vi "rs3 init devices_and_sensors.vi"(6 "rscontext":u64=1752067024, 8 "error in":errorcluster, 9 "api_version":i32=20710, 10 "Select Device":i32, 11 "Select Sensor":i32) -> (0 "error out":errorcluster, 1 "Adv. enable?":i32, 2 "init results":T3, 3 "init error":string, 4 "All Devices":T2(array[cluster]), 5 "Sensor Array":T1(array[cluster]), 7 "Found RealSense":bool)   [LabVIEW 2023]
doc: "Initialized the RealSense device. \nSelect the specific DEVICE and its specific SENSOR. \n\n\nINPUT:\nSelect Device The INDEX to the specific DEVICE handle\nSelect Sensor The INDEX to the specific SENSOR that is part of the selected DEVICE.\n \nOUTPUT:\ninit result Contains all the information about the selected device and its sensor. You will need to use the Dev Out HANDLE to communicate with the device. \n \nselected sensor array Contains the arrays of SENSORS attached to a specific DEVICE.\nall devices Contains array of all device that are attached to the PC."
panel:
  # "RS3 Init Device and Sensors"
  # "(C) Intel Corp. 2017,  AGJ"
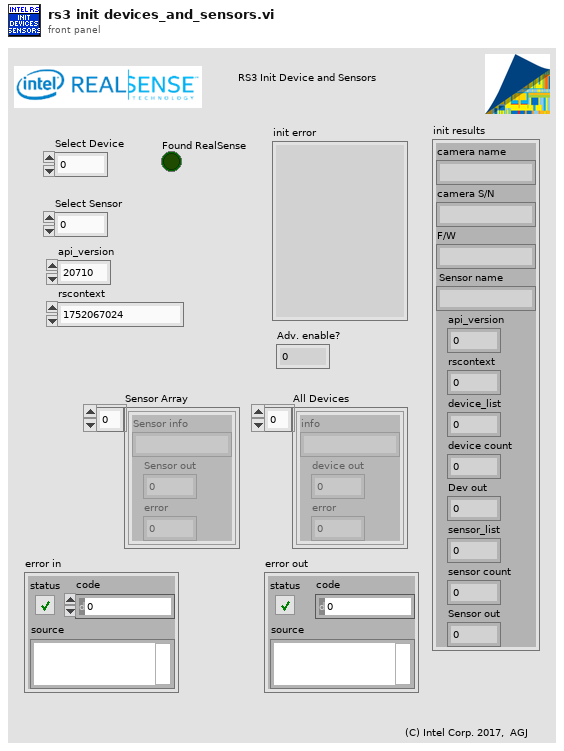
[diagram p1: front panel]
types:
  T1 = cluster{"Sensor info":string, "Sensor out":u64, "error":u64}[]
  T2 = cluster{"info":string, "device out":u64, "error":u64}[]
  T3 = cluster{"camera name":string, "camera S/N":string, "F/W":string, "Sensor name":string, "api_version":i32, "rscontext":u64, "device_list":u64, "device count":i32, "Dev out":u64, "sensor_list":u64, "sensor count":i32, "Sensor out":u64}
  T4 = cluster{"info":string, "device out":u64, "error":u64}
  T5 = cluster{"info":string, "info":string, "info":string, "Sensor info":string, "api_version":i32, "rscontext":u64, "device_list":u64, "device count":i32, "device out":u64, "sensor_list":u64, "sensor count":i32, "Sensor out":u64}
  T6 = cluster{"Sensor info":string, "Sensor out":u64, "error":u64}
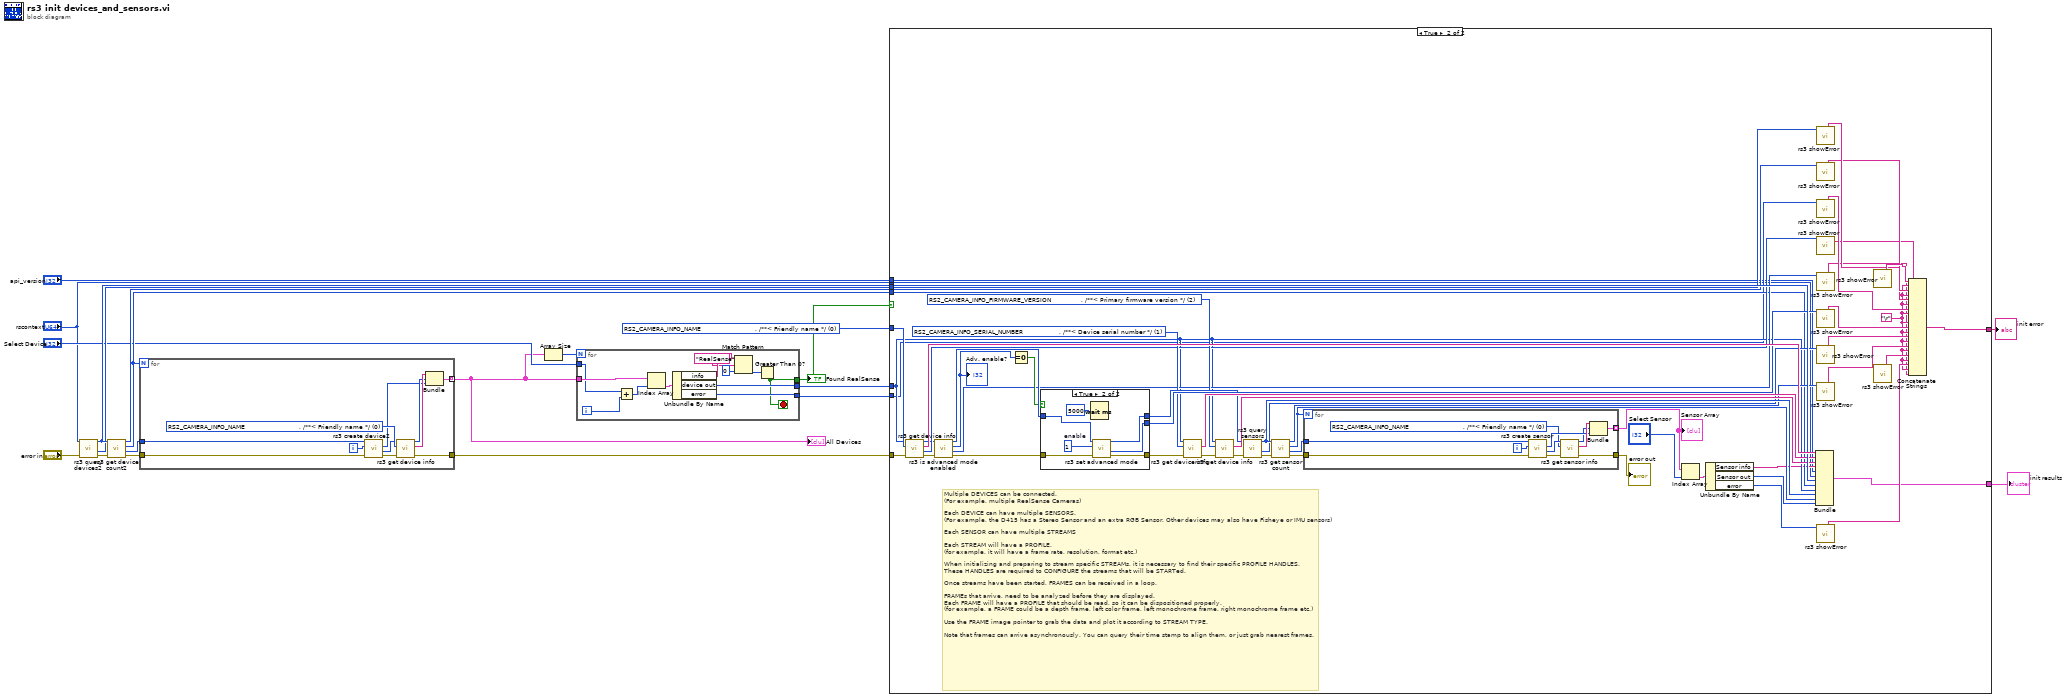
[diagram p0: block diagram]
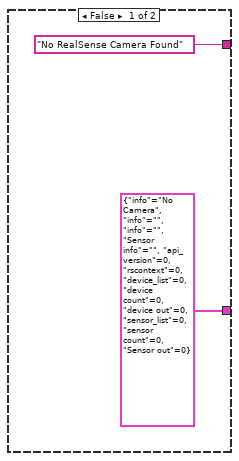
[diagram p2: hidden frame]
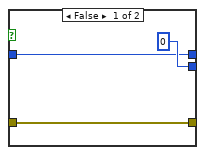
[diagram p3: hidden frame]
diagram:
  w19 = u16 0 items=["    RS2_CAMERA_INFO_NAME                           , /**< Friendly name */", "    RS2_CAMERA_INFO_SERIAL_NUMBER                  , /**< Device serial number */", "    RS2_CAMERA_INFO_FIRMWARE_VERSION               , /**< Primary firmware version */", "    RS2_CAMERA_INFO_PHYSICAL_PORT                       , /**< Unique identifier of the port the device is connected to (platform specific) */", "    RS2_CAMERA_INFO_DEBUG_OP_CODE                  , /**< If device supports firmware logging, this is the command to send to get logs from firmware */", "    RS2_CAMERA_INFO_ADVANCED_MODE                  , /**< True iff the device is in advanced mode */", "    RS2_CAMERA_INFO_PRODUCT_ID                     , /**< Product ID as reported in the USB descriptor */", "    RS2_CAMERA_INFO_CAMERA_LOCKED                  , /**< True iff EEPROM is locked */", "    RS2_CAMERA_INFO_COUNT                            /**< Number of enumeration values. Not a valid input: intended to be used in for-loops. */"] ("RS Camera info")
  n1 = call "rs3 query devices2.vi"("error in (no error)"="error in", "rscontext"="rscontext") -> ("error out"=w17:errorcluster, "error"=w16:u64, "device_list"=w20:u64)  [unwired: 7 in]
  n2 = call "rs3 get device count2.vi"("error in"=w17, "device"=w20) -> ("error out"=w11:errorcluster, "device list"=w14:u32, "device count"=w15:i32, "error"=w18:u64)  [unwired: 6 in]
  n3 = for {
    N: w15 -> [_]
    tunnel: w14 -> [w31]
    tunnel: [w25] -> w4 mode=indexing
    tunnel: w11 -> [w24]
    tunnel: [w23] -> w10
    i -> [w30]
    w28 = u16 0 items=["    RS2_CAMERA_INFO_NAME                           , /**< Friendly name */", "    RS2_CAMERA_INFO_SERIAL_NUMBER                  , /**< Device serial number */", "    RS2_CAMERA_INFO_FIRMWARE_VERSION               , /**< Primary firmware version */", "    RS2_CAMERA_INFO_PHYSICAL_PORT                       , /**< Unique identifier of the port the device is connected to (platform specific) */", "    RS2_CAMERA_INFO_DEBUG_OP_CODE                  , /**< If device supports firmware logging, this is the command to send to get logs from firmware */", "    RS2_CAMERA_INFO_ADVANCED_MODE                  , /**< True iff the device is in advanced mode */", "    RS2_CAMERA_INFO_PRODUCT_ID                     , /**< Product ID as reported in the USB descriptor */", "    RS2_CAMERA_INFO_CAMERA_LOCKED                  , /**< True iff EEPROM is locked */", "    RS2_CAMERA_INFO_COUNT                            /**< Number of enumeration values. Not a valid input: intended to be used in for-loops. */"] ("RS Camera info")
    n4 = call "rs3 create device2.vi"("error in (no error)"=w24, "Device index"=w30, "device list in"=w31) -> ("error out"=w29:errorcluster, "Dev out"=w22:u64, "error"=w21:u64)  [unwired: 5 in, 1 out]
    n5 = call "rs3 get device info.vi"("error in (no error)"=w29, "RS Camera info"=w28, "device in"=w22) -> ("error out"=w23:errorcluster, "info"=w27:string, "device out"=w26:u64)  [unwired: 5 in, 1 out]
    n6 = Bundle("info"=w27, "device out"=w26, "error"=w21) -> (w25:T4)  [unwired: 1 in]
  }
  "All Devices" <- w4
  n7 = Array Size(array=w4) -> (size(s)=w5:i32)
  n8 = for {
    N: w5 -> [_]
    tunnel: w4 -> [w43]
    tunnel: "Select Device" -> [w34]
    tunnel: [w41] -> w12
    tunnel: [w40] -> w9
    tunnel: [w32] -> w8
    i -> [w35]
    stop <- w32 stop-if-true
    n9 = Add(x=w34, y=w35) -> (x+y=w36:i32)
    n10 = Index Array(array=w43, index=w36) -> (element=w42:T4)
    n11 = Unbundle By Name(w42) -> ("info"=w38:string, "device out"=w41:u64, "error"=w40:u64)
    n12 = Match Pattern(string=w38, regular expression="RealSense" ("string"), offset (0)=0) -> (offset past match=w33:i32)  [unwired: 3 out]
    n13 = Greater Than 0?(x=w33) -> (x > 0?=w32:bool)
  }
  "Found RealSense" <- w8
  n14 = case shown="True" w8 {
    tunnel: w20 -> [_ w99]
    tunnel: w19 -> [_ w86]
    tunnel: w18 -> [_ w84]
    tunnel: w16 -> [_ w83]
    tunnel: w15 -> [_ w63]
    tunnel: w12 -> [_ w62]
    tunnel: w10 -> [_ w61]
    tunnel: w9 -> [_ w60]
    tunnel: "rscontext" -> [_ w49]
    tunnel: "api_version" -> [_ w48]
    tunnel: ["No RealSense Camera Found" w47] -> w7
    tunnel: [T5 {"info"="No Camera", "info"="", "info"="", "Sensor info"="", "api_version"=0, "rscontext"=0, "device_list"=0, "device count"=0, "device out"=0, "sensor_list"=0, "sensor count"=0, "Sensor out"=0} w46] -> w6
    frame False {
    }
    frame True {
      w65 = "\r"
      w93 = u16 2 items=["    RS2_CAMERA_INFO_NAME                           , /**< Friendly name */", "    RS2_CAMERA_INFO_SERIAL_NUMBER                  , /**< Device serial number */", "    RS2_CAMERA_INFO_FIRMWARE_VERSION               , /**< Primary firmware version */", "    RS2_CAMERA_INFO_PHYSICAL_PORT                       , /**< Unique identifier of the port the device is connected to (platform specific) */", "    RS2_CAMERA_INFO_DEBUG_OP_CODE                  , /**< If device supports firmware logging, this is the command to send to get logs from firmware */", "    RS2_CAMERA_INFO_ADVANCED_MODE                  , /**< True iff the device is in advanced mode */", "    RS2_CAMERA_INFO_PRODUCT_ID                     , /**< Product ID as reported in the USB descriptor */", "    RS2_CAMERA_INFO_CAMERA_LOCKED                  , /**< True iff EEPROM is locked */", "    RS2_CAMERA_INFO_COUNT                            /**< Number of enumeration values. Not a valid input: intended to be used in for-loops. */"] ("RS Camera info")
      w92 = u16 1 items=["    RS2_CAMERA_INFO_NAME                           , /**< Friendly name */", "    RS2_CAMERA_INFO_SERIAL_NUMBER                  , /**< Device serial number */", "    RS2_CAMERA_INFO_FIRMWARE_VERSION               , /**< Primary firmware version */", "    RS2_CAMERA_INFO_PHYSICAL_PORT                       , /**< Unique identifier of the port the device is connected to (platform specific) */", "    RS2_CAMERA_INFO_DEBUG_OP_CODE                  , /**< If device supports firmware logging, this is the command to send to get logs from firmware */", "    RS2_CAMERA_INFO_ADVANCED_MODE                  , /**< True iff the device is in advanced mode */", "    RS2_CAMERA_INFO_PRODUCT_ID                     , /**< Product ID as reported in the USB descriptor */", "    RS2_CAMERA_INFO_CAMERA_LOCKED                  , /**< True iff EEPROM is locked */", "    RS2_CAMERA_INFO_COUNT                            /**< Number of enumeration values. Not a valid input: intended to be used in for-loops. */"] ("RS Camera info")
      # "Multiple DEVICES can be connected. \n(For example, multiple RealSense Cameras)\n\nEach DEVICE can have multiple SENSORS. \n(For example, the D415 has a Stereo Sensor and an extra RGB Sensor. Other devices may also have Fisheye or IMU sensors) \n\nEach SENSOR can have multiple STREAMS\n\nEach STREAM will have a PROFILE. \n(for example, it will have a frame rate, resolution, format etc.)\n\nWhen initializing and preparing to stream specific STREAMs, it is necessary to find their specific PROFILE HANDLES.\nThese HANDLES are required to CONFIGURE the streams that will be STARTed. \n\nOnce streams have been started, FRAMES can be received in a loop. \n \nFRAMEs that arrive, need to be analyzed before they are displayed. \nEach FRAME will have a PROFILE that should be read, so it can be dispositioned properly.\n(for example, a FRAME could be a depth frame, left color frame, left monochrome frame, right monochrome frame etc.)\n\nUse the FRAME image pointer to grab the data and plot it according to STREAM TYPE.\n\nNote that frames can arrive asynchronously. You can query their time stamp to align them, or just grab nearest frames."
      n15 = call "rs3 get device info.vi"("error in (no error)"=w61, "RS Camera info"=w86, "device in"=w62) -> ("error out"=w72:errorcluster, "error"=w85:u64, "info"=w100:string, "device out"=w70:u64)  [unwired: 5 in]
      n16 = call "rs3 is advanced mode enabled.vi"("error in (no error)"=w72, "device in"=w70) -> ("error out"=w71:errorcluster, "error"=w66:u64, "enable?"=w68:i32, "device out"=w69:u64)  [unwired: 6 in]
      "Adv. enable?" <- w68
      n17 = Equal To 0?(x=w68) -> (x = 0?=w67:bool)
      n18 = case shown="True" w67 {
        tunnel: [u64 0 ("error") w122] -> w96
        tunnel: [w113 w120] -> w95
        tunnel: w69 -> [w113 w119]
        tunnel: [w115 w118] -> w94
        tunnel: w71 -> [w115 w117]
        frame False {
        }
        frame True {
          w121 = 1  # enable
          n19 = Wait (ms)(milliseconds to wait=u32 5000) -> ()  [unwired: 1 out]
          n20 = call "rs3 set advanced mode.vi"("error in (no error)"=w117, "enable"=w121, "device in"=w119) -> ("error out"=w118:errorcluster, "error"=w122:u64, "device out"=w120:u64)  [unwired: 6 in]
        }
      }
      n21 = call "rs3 get device info.vi"("error in (no error)"=w94, "RS Camera info"=w92, "device in"=w62) -> ("error out"=w90:errorcluster, "info"=w97:string)  [unwired: 5 in, 2 out]
      n22 = call "rs3 get device info.vi"("error in (no error)"=w90, "RS Camera info"=w93, "device in"=w62) -> ("error out"=w91:errorcluster, "info"=w98:string)  [unwired: 5 in, 2 out]
      n23 = call "rs3 query sensors.vi"("error in (no error)"=w91, "device in"=w95) -> ("error out"=w88:errorcluster, "error"=w87:u64, "sensor_list"=w101:u64)  [unwired: 7 in]
      n24 = call "rs3 get sensor count.vi"("error in"=w88, "sensor_list"=w101) -> ("error out"=w58:errorcluster, "sensor_list_out"=w57:u64, "sensor count"=w59:i32, "error"=w89:u64)  [unwired: 6 in]
      n25 = for {
        N: w59 -> [_]
        tunnel: w58 -> [w112]
        tunnel: w57 -> [w109]
        tunnel: [w103] -> w56 mode=indexing
        tunnel: [w102] -> w51
        i -> [w110]
        w105 = u16 0 items=["    RS2_CAMERA_INFO_NAME                           , /**< Friendly name */", "    RS2_CAMERA_INFO_SERIAL_NUMBER                  , /**< Device serial number */", "    RS2_CAMERA_INFO_FIRMWARE_VERSION               , /**< Primary firmware version */", "    RS2_CAMERA_INFO_PHYSICAL_PORT                       , /**< Unique identifier of the port the device is connected to (platform specific) */", "    RS2_CAMERA_INFO_DEBUG_OP_CODE                  , /**< If device supports firmware logging, this is the command to send to get logs from firmware */", "    RS2_CAMERA_INFO_ADVANCED_MODE                  , /**< True iff the device is in advanced mode */", "    RS2_CAMERA_INFO_PRODUCT_ID                     , /**< Product ID as reported in the USB descriptor */", "    RS2_CAMERA_INFO_CAMERA_LOCKED                  , /**< True iff EEPROM is locked */", "    RS2_CAMERA_INFO_COUNT                            /**< Number of enumeration values. Not a valid input: intended to be used in for-loops. */"] ("RS Sensor info")
        n26 = call "rs3 create sensor.vi"("error in (no error)"=w112, "Sensor index"=w110, "Sensor list"=w109) -> ("error out"=w111:errorcluster, "Sensor out"=w107:u64, "error"=w106:u64)  [unwired: 5 in, 1 out]
        n27 = call "rs3 get sensor info.vi"("error in (no error)"=w111, "RS Camera info"=w105, "Sensor in"=w107) -> ("error out"=w102:errorcluster, "Sensor info"=w108:string, "Sensor out"=w104:u64)  [unwired: 5 in, 1 out]
        n28 = Bundle("Sensor info"=w108, "Sensor out"=w104, "error"=w106) -> (w103:T6)  [unwired: 1 in]
      }
      "error out" <- w51
      "Sensor Array" <- w56
      n29 = Index Array(array=w56, index="Select Sensor") -> (element=w54:T6)
      n30 = Unbundle By Name(w54) -> ("Sensor info"=w50:string, "Sensor out"=w53:u64, "error"=w52:u64)
      n31 = Bundle("info"=w100, "info"=w97, "info"=w98, "Sensor info"=w50, "api_version"=w48, "rscontext"=w49, "device_list"=w99, "device count"=w63, "device out"=w62, "sensor_list"=w101, "sensor count"=w59, "Sensor out"=w53) -> (w46:T5)  [unwired: 1 in]
      n32 = call "rs3 showError.vi"("error"=w83) -> ("Error summary"=w81:string)  [unwired: 6 in, 4 out]
      n33 = call "rs3 showError.vi"("error"=w84) -> ("Error summary"=w80:string)  [unwired: 6 in, 4 out]
      n34 = call "rs3 showError.vi"("error"=w60) -> ("Error summary"=w79:string)  [unwired: 6 in, 4 out]
      n35 = call "rs3 showError.vi"("error"=w85) -> ("Error summary"=w78:string)  [unwired: 6 in, 4 out]
      n36 = call "rs3 showError.vi"("error"=w66) -> ("Error summary"=w64:string)  [unwired: 6 in, 4 out]
      n37 = call "rs3 showError.vi"("error"=w96) -> ("Error summary"=w77:string)  [unwired: 6 in, 4 out]
      n38 = call "rs3 showError.vi"("error"=w87) -> ("Error summary"=w76:string)  [unwired: 6 in, 4 out]
      n39 = call "rs3 showError.vi"("error"=w89) -> ("Error summary"=w75:string)  [unwired: 6 in, 4 out]
      n40 = call "rs3 showError.vi"("error"=w52) -> ("Error summary"=w73:string)  [unwired: 6 in, 4 out]
      n41 = call "rs3 showError.vi"() -> ("Error summary"=w82:string)  [unwired: 7 in, 4 out]
      n42 = call "rs3 showError.vi"() -> ("Error summary"=w74:string)  [unwired: 7 in, 4 out]
      n43 = Concatenate Strings(w82, w65, w81, w65, w80, w65, w79, w65, w78, w65, w77, w65, w76, w65, w75, w65, w74, w65, w73, w65, w64) -> (w47:string)
    }
  }
  "init error" <- w7
  "init results" <- w6
